vi "Match Asterisk Pattern.vi"(0 "String":string, 2 "* Expression":string) -> (6 "String (Dup)":string, 10 "Matched":bool)   [LabVIEW 2017, in "CSM Shared.lvlib"]
uses:
  CSM Shared.lvlib
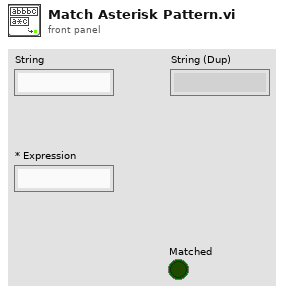
[diagram p1: front panel]
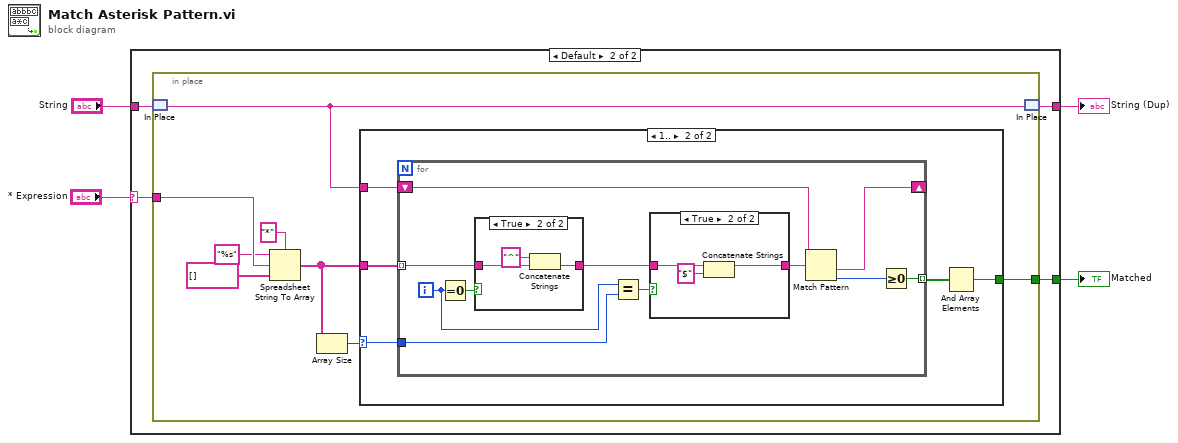
[diagram p0: block diagram]
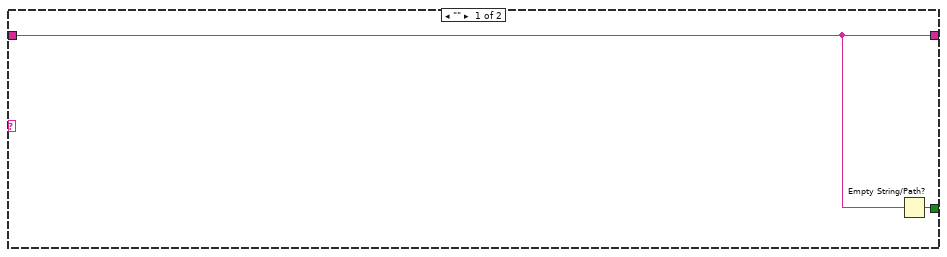
[diagram p2: hidden frame]
diagram:
  n1 = case shown="Default" "* Expression" {
    selector: "* Expression" -> [_ w10]
    tunnel: "String" -> [w5 w8]
    tunnel: [w6 w9] -> w2
    tunnel: [w5 w7] -> w1
    frame "" {
      n2 = Empty String/Path?(string/path=w5) -> (empty?=w6:bool)
    }
    frame Default {
      n3 = in-place {
        in-place-border: w10 -> [w18]
        in-place-border: [w12] -> w9
        n4 = in-place-match #1(w8) -> (w11:string)
        n5 = Spreadsheet String To Array(delimiter (Tab)="*", format string="%s", spreadsheet string=w18, array type (2D Dbl)=string[] [] ("Array of Strings")) -> (array=w13:string[])
        n6 = Array Size(array=w13) -> (size(s)=w14:i32)
        n7 = case shown="1.." w14 {
          selector: w14 -> [_ w19]
          tunnel: w11 -> [_ w23]
          tunnel: w13 -> [_ w22]
          tunnel: [_ w20] -> w12
          frame 0, Default {
          }
          frame 1.. {
            n8 = for {
              tunnel: w22 -> [w30] mode=indexing
              shift-right: [w33] -> _
              shift-left: w23 -> [w34]
              tunnel: [w31] -> w21 mode=indexing
              tunnel: w19 -> [w27]
              i -> [w28]
              n9 = Equal To 0?(x=w28) -> (x = 0?=w29:bool)
              n10 = case shown="True" w29 {
                tunnel: [w39 w41] -> w25
                tunnel: w30 -> [w39 w42]
                frame False {
                }
                frame True {
                  n11 = Concatenate Strings("^" ("string"), w42) -> (w41:string)
                }
              }
              n12 = Equal?(x=w28, y=w27) -> (x = y?=w26:bool)
              n13 = case shown="True" w26 {
                tunnel: w25 -> [w35 w38]
                tunnel: [w35 w37] -> w24
                frame False {
                }
                frame True {
                  n14 = Concatenate Strings(w38, "$" ("string")) -> (w37:string)
                }
              }
              n15 = Match Pattern(string=w34, regular expression=w24) -> (after substring=w33:string, offset past match=w32:i32)  [unwired: 1 in, 2 out]
              n16 = Greater Or Equal To 0?(x=w32) -> (x >= 0?=w31:bool)
            }
            n17 = And Array Elements(Boolean array=w21) -> (logical AND=w20:bool)
          }
        }
        n18 = in-place-match #1(w11) -> (w7:string)
      }
    }
  }
  "String (Dup)" <- w1
  "Matched" <- w2
